vi "Write to List.vi"(9 "Publication Time":timestamp, 10 "Value to Publish":variant, 11 "Topic in":refnum<class "Topic.lvclass">) -> (3 "Topic out":refnum<class "Topic.lvclass">)   [LabVIEW 2017, in "Mediator.lvlib" / "Topic.lvclass"]
uses:
  Topic.lvclass
  Topic.lvclass/Topic.ctl
  IMediator/ISubscriptionPolicy/ISubscriptionPolicy Reference.ctl
  IMediator/ISubscriptionPolicy/ISubscriptionPolicy.lvclass
  IMediator/ISubscriptionPolicy/ISubscriptionPolicy.lvclass/ISubscriptionPolicy.ctl
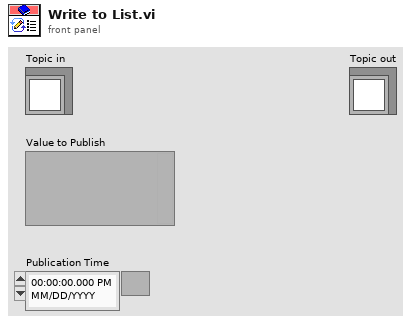
[diagram p1: front panel]
types:
  T1 = typedef "IMediator.lvlib/ISubscriptionPolicy.lvclass/ISubscriptionPolicy Reference.ctl" = refnum<data-value>
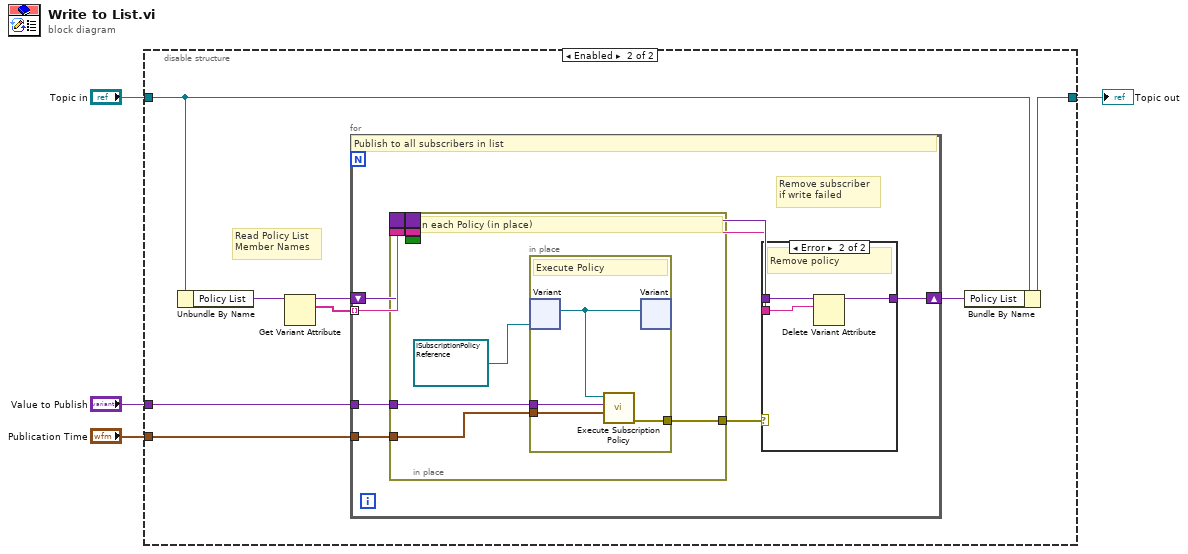
[diagram p0: block diagram]
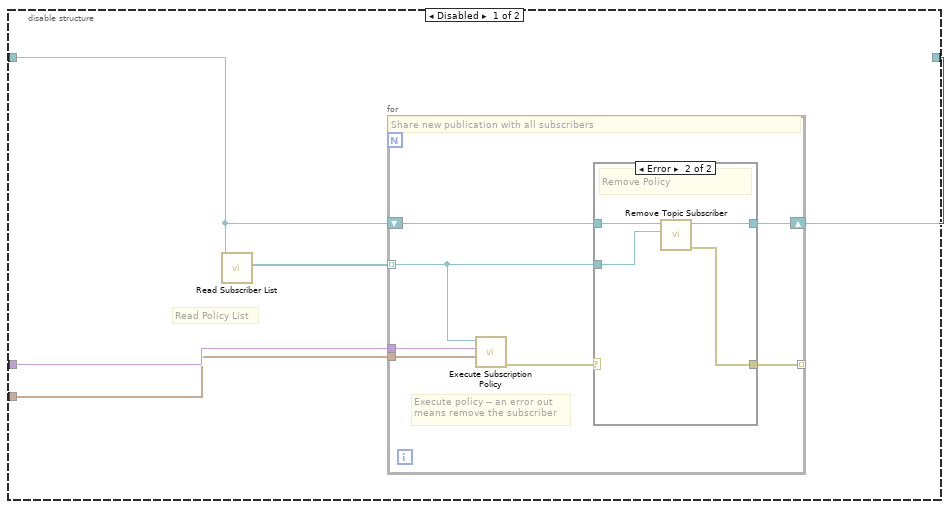
[diagram p2: hidden frame]
diagram:
  n1 = disable-structure shown="Enabled" {
    disable-tunnel: [w9 w25] -> w1
    disable-tunnel: "Topic in" -> [w7 w28]
    disable-tunnel: "Value to Publish" -> [w6 w31]
    disable-tunnel: "Publication Time" -> [w5 w30]
    frame Disabled {
      # "Read Policy List"
      n2 = call "Read Subscriber List.vi"("Topic in"=w7) -> ("Subscriber Policy List"=w8:T1[])  [unwired: 10 in]
      n3 = for {
        tunnel: w8 -> [w11] mode=indexing
        tunnel: w6 -> [w16]
        tunnel: [w17] -> w10 mode=indexing
        tunnel: w5 -> [w12]
        shift-right: [w14] -> w9
        shift-left: w7 -> [w15]
        # "Execute policy -- an error out\nmeans remove the subscriber"
        # "Share new publication with all subscribers"
        n4 = call "Execute Subscription Policy.vi"("Publish Time"=w12, "New Topic Value"=w16, "Subscription Policy"=w11) -> ("error out (Unsubscribe?)"=w13:errorcluster)  [unwired: 8 in]
        n5 = case shown="Error" w13 {
          selector: w13 -> [w18 _]
          tunnel: [w18 w23] -> w17
          tunnel: w15 -> [w19 w22]
          tunnel: [w19 w21] -> w14
          tunnel: w11 -> [_ w20]
          frame No Error {
            # "Write OK"
          }
          frame Error {
            # "Remove Policy"
            n6 = call "Remove Topic Subscriber.vi"("Subscription Policy"=w20, "Topic in"=w22) -> ("error out"=w23:errorcluster, "Topic out"=w21:refnum<class "Topic.lvclass">)  [unwired: 8 in]
          }
        }
      }
    }
    frame Enabled {
      # "Read Policy List\nMember Names"
      n7 = Unbundle By Name(w28) -> ("Policy List"=w27:variant)
      n8 = Get Variant Attribute(Variant=w27) -> (duplicate Variant=w26:variant, names=w29:string[])  [unwired: 3 in, 2 out]
      n9 = for {
        tunnel: w31 -> [w39]
        tunnel: w30 -> [w38]
        shift-right: [w33] -> w24
        shift-left: w26 -> [w36]
        tunnel: w29 -> [w37] mode=indexing
        # "Remove subscriber\nif write failed"
        # "Publish to all subscribers in list"
        n10 = in-place {
          in-place-border: [w44] -> w34
          in-place-border: w39 -> [w49]
          in-place-border: w38 -> [w48]
          border: w36 -> [_]
          border: w37 -> [_]
          border: [_] -> w35
          border: [_] -> w32
          border: _ -> [_]
          # "Obtain each Policy (in place)"
          n11 = in-place {
            in-place-border: [w53] -> w44
            in-place-border: w49 -> [w52]
            in-place-border: w48 -> [w51]
            # "Execute Policy"
            n12 = in-place-variant #1(w47, T1 refnum ("Subscription Policy")) -> (w50:T1)  [unwired: 1 out]
            n13 = call "Execute Subscription Policy.vi"("Publish Time"=w51, "New Topic Value"=w52, "Subscription Policy"=w50) -> ("error out (Unsubscribe?)"=w53:errorcluster)  [unwired: 8 in]
            n14 = in-place-variant #1(w50) -> (w45:variant)  [unwired: 1 out]
          }
        }
        n15 = case shown="Error" w34 {
          tunnel: w35 -> [w40 w43]
          tunnel: [w40 w42] -> w33
          tunnel: w32 -> [_ w41]
          frame No Error {
            # "Write OK"
          }
          frame Error {
            # "Remove policy"
            n16 = Delete Variant Attribute(6:w41, 7:w43) -> (3:w42:variant)  [unwired: 1 in, 2 out]
          }
        }
      }
      n17 = Bundle By Name(cluster=w28, "Policy List"=w24) -> (w25:refnum<class "Topic.lvclass">)
    }
  }
  "Topic out" <- w1
